vi "Velocity_Trajectory.vi"() -> ()   [LabVIEW 2017]
panel:
  out "Velocity Profile":dbl[](graph)
  in  "Max Velocity":dbl
  in  "Theta Final":dbl
  in  "Theta Initial":dbl
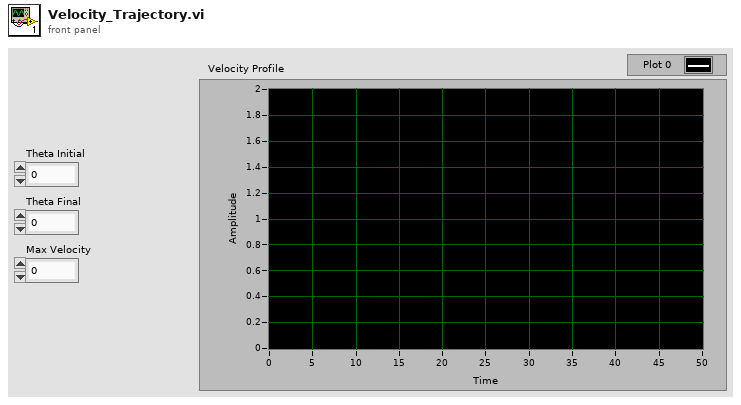
[diagram p1: front panel]
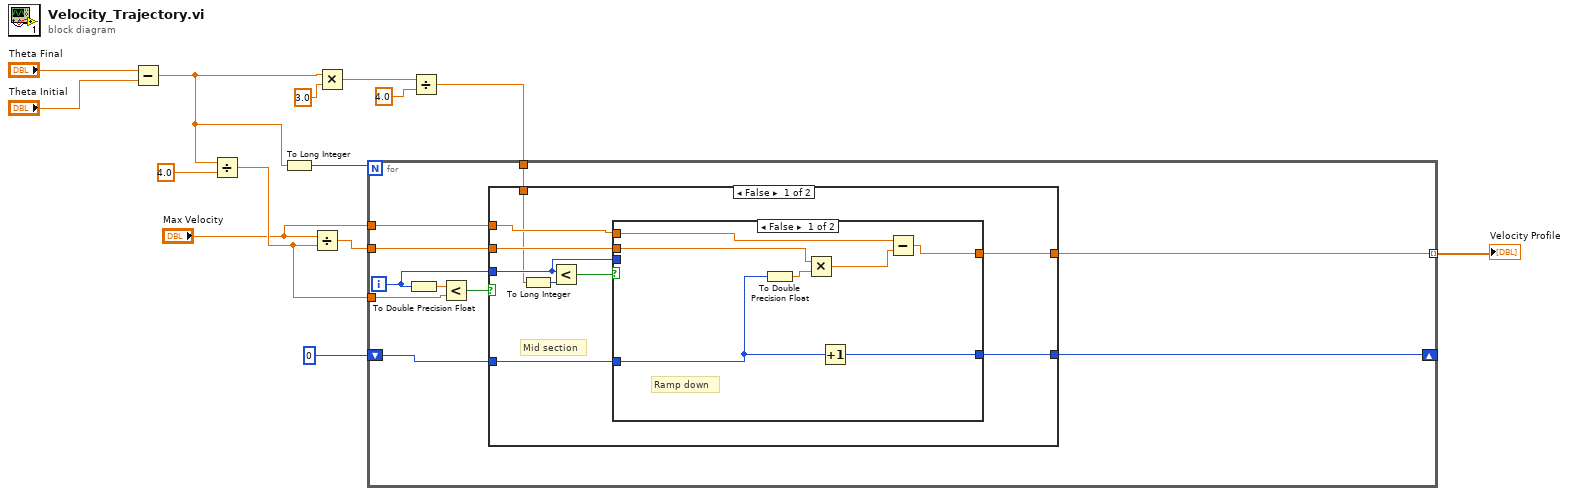
[diagram p0: block diagram]
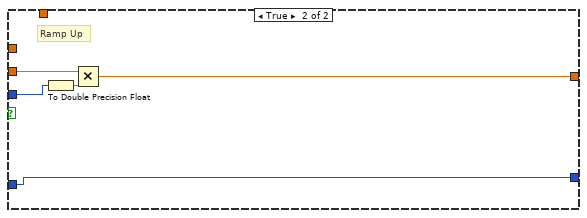
[diagram p3: hidden frame]
diagram:
  n1 = Subtract(x="Theta Final", y="Theta Initial") -> (x-y=w7:dbl)
  n2 = Divide(x=w7, y=4.0) -> (x/y=w6:dbl)
  n3 = To Long Integer(number=w7) -> (32bit integer=w1:i32)
  n4 = Divide(x="Max Velocity", y=w6) -> (x/y=w8:dbl)
  n5 = Multiply(x=w7, y=3.0) -> (x*y=w10:dbl)
  n6 = Divide(x=w10, y=4.0) -> (x/y=w5:dbl)
  n7 = for {
    N: w1 -> [_]
    tunnel: w8 -> [w22]
    tunnel: w6 -> [w23]
    tunnel: [w21] -> w3 mode=indexing
    tunnel: w5 -> [w20]
    tunnel: "Max Velocity" -> [w19]
    shift-right: [w17] -> _
    shift-left: 0 -> [w18]
    i -> [w16]
    n8 = To Double Precision Float(number=w16) -> (double precision float=w15:dbl)
    n9 = Less?(x=w15, y=w23) -> (x < y?=w24:bool)
    n10 = case shown="False" w24 {
      tunnel: w22 -> [w32 w47]
      tunnel: [w31 w46] -> w21
      tunnel: w20 -> [w26 _]
      tunnel: w19 -> [w30 _]
      tunnel: w16 -> [w29 w43]
      tunnel: w18 -> [w28 w45]
      tunnel: [w27 w45] -> w17
      frame False {
        # "Mid section"
        n11 = To Long Integer(number=w26) -> (32bit integer=w25:i32)
        n12 = Less?(x=w29, y=w25) -> (x < y?=w33:bool)
        n13 = case shown="False" w33 {
          tunnel: w32 -> [w34 _]
          tunnel: [w37 w42] -> w31
          tunnel: w30 -> [w38 w42]
          tunnel: w29 -> [_ _]
          tunnel: w28 -> [w39 w41]
          tunnel: [w40 w41] -> w27
          frame False {
            # "Ramp down"
            n14 = To Double Precision Float(number=w39) -> (double precision float=w36:dbl)
            n15 = Multiply(x=w34, y=w36) -> (x*y=w35:dbl)
            n16 = Increment(x=w39) -> (x+1=w40:i32)
            n17 = Subtract(x=w38, y=w35) -> (x-y=w37:dbl)
          }
          frame True {
          }
        }
      }
      frame True {
        # "Ramp Up"
        # "Ramp Up"
        n18 = To Double Precision Float(number=w43) -> (double precision float=w44:dbl)
        n19 = Multiply(x=w47, y=w44) -> (x*y=w46:dbl)
      }
    }
  }
  "Velocity Profile" <- w3
